vi "Open_Top_Level_VIs.vi"(8 "error in (no error)":errorcluster, 11 "Build in":refnum<class "AB_PackedLibrary.lvclass">) -> (0 "error out":errorcluster, 2 "Top-Level VIs":refnum<vi>[](array[refnum]), 3 "Build out":refnum<class "AB_PackedLibrary.lvclass">)   [LabVIEW 2020, in "AB_PackedLibrary.lvclass"]
uses:
  <vilib>/AppBuilder/AB_Classes/PackedLib/AB_PackedLibrary.lvclass
  <resource>/Framework/Providers/Common/provcom_StringGlobals.vi
  <vilib>/AppBuilder/AB_Classes/TargetFile/AB_Targetfile.lvclass
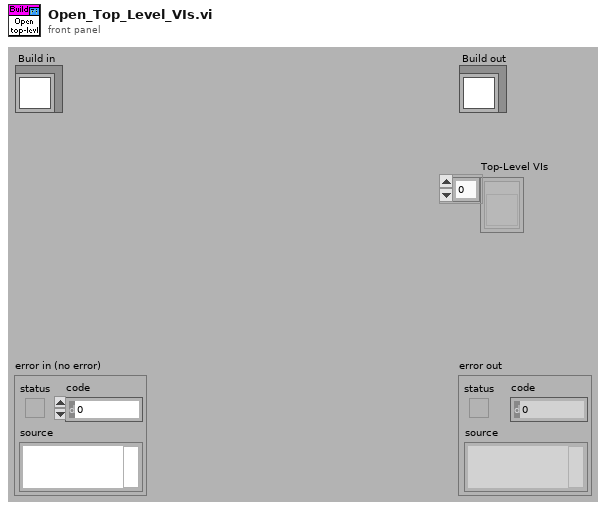
[diagram p1: front panel]
types:
  T1 = enum32{"invalid scope", "public", "private", "protected", "community"}
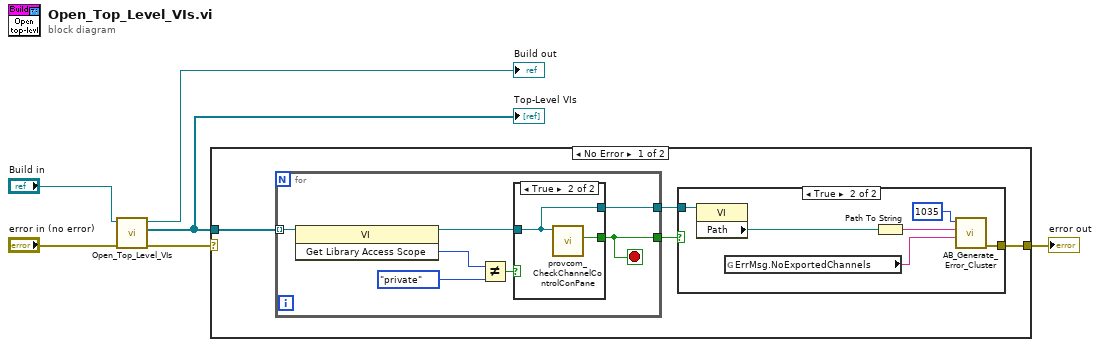
[diagram p0: block diagram]
diagram:
  n1 = call-parent "Open_Top_Level_VIs.vi"("error in (no error)"="error in (no error)", "Build in"="Build in") -> ("error out"=w3:errorcluster, "Top-Level VIs"=w1:refnum<vi>[], "Build out"=→"Build out":refnum<class "AB_PackedLibrary.lvclass">)  [unwired: 7 in]
  "Top-Level VIs" <- w1
  n2 = case shown="No Error" w3 {
    selector: w3 -> [_ w27]
    tunnel: w1 -> [w7 _]
    tunnel: [w8 w27] -> w2
    frame No Error {
      n3 = for {
        tunnel: w7 -> [w20] mode=indexing
        tunnel: [w23] -> w10
        tunnel: [w17] -> w9
        stop <- w23 stop-if-true
        n4 = invoke class="VI" method="Get Library Access Scope"(reference=w20) -> (reference out=w19:refnum<vi>, "Get Library Access Scope"=w22:T1)  [unwired: 2 in, 1 out]
        n5 = Not Equal?(x=w22, y=T1."private") -> (x != y?=w18:bool)
        n6 = case shown="True" w18 {
          tunnel: [_ w26] -> w23
          tunnel: w19 -> [w24 w25]
          tunnel: [w24 w25] -> w17
          frame False {
          }
          frame True {
            n7 = call <resource>:"provcom_CheckChannelControlConPane.vi"("VI Refnum"=w25) -> ("Channel Control?"=w26:bool)  [unwired: 1 in, 9 out]
          }
        }
      }
      n8 = case shown="True" w10 {
        tunnel: w9 -> [_ w13]
        tunnel: [_ w11] -> w8
        frame False {
        }
        frame True {
          n9 = property class="VI"(reference=w13) -> ("Path"=w15:path)  [unwired: 1 in, 2 out]
          n10 = global read "provcom_StringGlobals.vi" "ErrMsg.NoExportedChannels"() -> (w12:string)
          n11 = Path To String(path=w15) -> (string=w14:string)
          n12 = call <vilib>:"AB_Generate_Error_Cluster.vi"("Additional Message"=w12, "source"=w14, "Code"=1035) -> ("error out"=w11:errorcluster)  [unwired: 1 in, 7 out]
        }
      }
    }
    frame Error {
    }
  }
  "error out" <- w2
